vi "Write ALID.vi"(8 "error in (no error)":errorcluster, 10 "ALID":u32, 11 "11-Alarm Management in":refnum<class "11-Alarm Management.lvclass">) -> (0 "error out":errorcluster, 3 "11-Alarm Management out":refnum<class "11-Alarm Management.lvclass">)   [LabVIEW 2020, in "SECS Scenarios.lvlib" / "11-Alarm Management.lvclass"]
uses:
  11-Alarm Management.lvclass
  11-Alarm Management.lvclass/11-Alarm Management.ctl
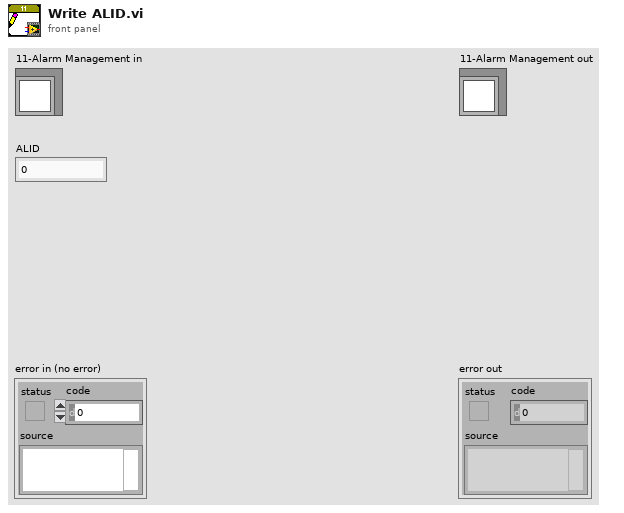
[diagram p1: front panel]
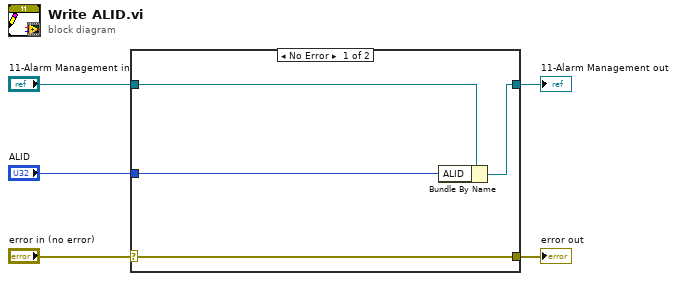
[diagram p0: block diagram]
diagram:
  n1 = case shown="No Error" "error in (no error)" {
    selector: "error in (no error)" -> [w9 w10]
    tunnel: [w9 w10] -> w4
    tunnel: [w7 w11] -> w2
    tunnel: "11-Alarm Management in" -> [w8 w11]
    tunnel: "ALID" -> [w6 _]
    frame No Error {
      n2 = Bundle By Name(cluster=w8, "ALID"=w6) -> (w7:refnum<class "11-Alarm Management.lvclass">)
    }
    frame Error {
    }
  }
  "error out" <- w4
  "11-Alarm Management out" <- w2
